vi "create_base_path.vi"(1 "project name":string) -> (0 "base path":path)   [LabVIEW 2018]
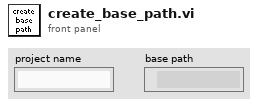
[diagram p1: front panel]
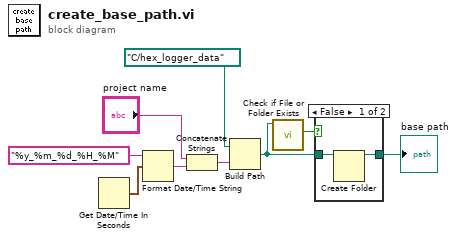
[diagram p0: block diagram]
diagram:
  n1 = Get Date/Time In Seconds() -> (seconds since 1Jan1904=w2:timestamp)
  n2 = Format Date/Time String(time format string (%c)="%y_%m_%d_%H_%M", seconds (now)=w2) -> (date/time string=w4:string)  [unwired: 1 in]
  n3 = Concatenate Strings("project name", w4) -> (w5:string)
  n4 = Build Path(base path=path "C:/hex_logger_data", name or relative path=w5) -> (appended path=w7:path)
  n5 = call <vilib>:"Check if File or Folder Exists.vi"("path"=w7) -> ("file or folder exists?"=w8:bool)  [unwired: 8 in, 2 out]
  n6 = case shown="False" w8 {
    tunnel: [w10 w12] -> w6
    tunnel: w7 -> [w11 w12]
    frame False {
      n7 = Create Folder(path (use dialog)=w11) -> (created path=w10:path)  [unwired: 2 in, 2 out]
    }
    frame True {
    }
  }
  "base path" <- w6
